vi "GetPropertyAbstract.vi"(8 "error in (no error)":errorcluster, 11 "reference in":refnum<class "G#MethodTemplates.lvclass">) -> (0 "error out":errorcluster, 2 "Numeric":dbl, 3 "reference out":refnum<class "G#MethodTemplates.lvclass">)   [LabVIEW 2017, in "G#MethodTemplates.lvclass"]
uses:
  <vilib>/addons/_AddQ/G#Templates/G#MethodTemplates/G#MethodTemplates.lvclass
  C:/Program Files (x86)/National Instruments/LabVIEW 2017/vi.lib/addons/_AddQ/G#Object/G#Object.lvclass
  <vilib>/addons/_AddQ/G#Object/G#Object.lvclass
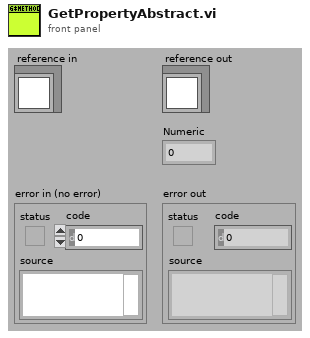
[diagram p1: front panel]
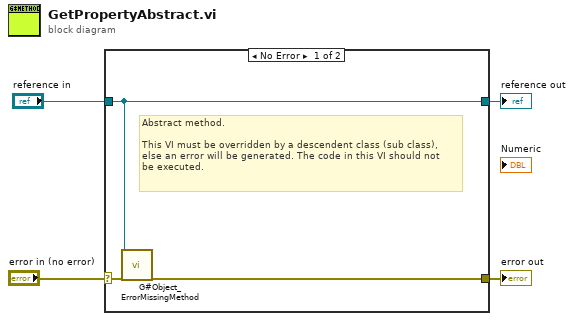
[diagram p0: block diagram]
diagram:
  n1 = case shown="No Error" "error in (no error)" {
    selector: "error in (no error)" -> [w6 w9]
    tunnel: [w5 w9] -> w3
    tunnel: [w7 w8] -> w1
    tunnel: "reference in" -> [w7 w8]
    frame No Error {
      # "Abstract method.\n\nThis VI must be overridden by a descendent class (sub class),\nelse an error will be generated. The code in this VI should not\nbe executed."
      n2 = call <vilib>:"G#Object_ErrorMissingMethod.vi"("reference in"=w7, "error in (no error)"=w6) -> ("error out"=w5:errorcluster)  [unwired: 16 in, 1 out]
    }
    frame Error {
    }
  }
  "error out" <- w3
  "reference out" <- w1
